vi "tsapp_configure_baudrate_can.vi"(5 "AInstallTermResistor120Ohm":bool, 7 "AListenOnly":bool, 8 "error in (no error)":errorcluster caption="错误输入（无错误）", 9 "ABaudrateKbps":sgl, 10 "AIdxChn":i32, 11 "路径输入":path) -> (0 "error out":errorcluster caption="错误输出", 2 "return":i32, 3 "路径输出":path)   [LabVIEW 2014]
doc: "Function Introduction ：\nSet parameters such as baud rate for CAN channel\nCall location ：\nBefore connecting hardware devices, set the parameters of the channel first\ninput parameter ：\nAIdxChn: Application Channel Number\nABaud rate Kbps: baud rate (kbps)\nAListenOnly: Whether to only listen mode, if enabled, can only receive data\nAInstallTermResistor120Ohm: Can only internal terminal resistors of the device be used\nReturn value ：\n==0: Connection successful\nOther: Check for error codes"
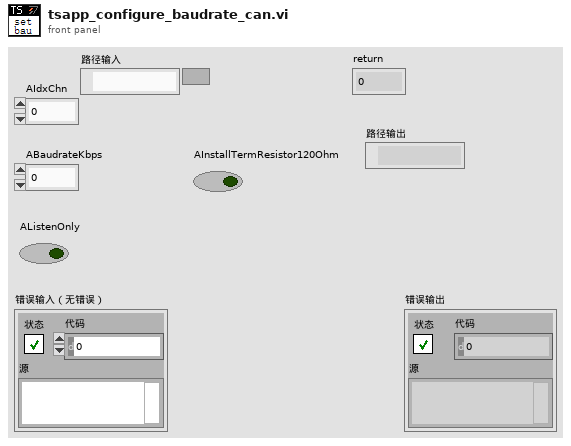
[diagram p1: front panel]
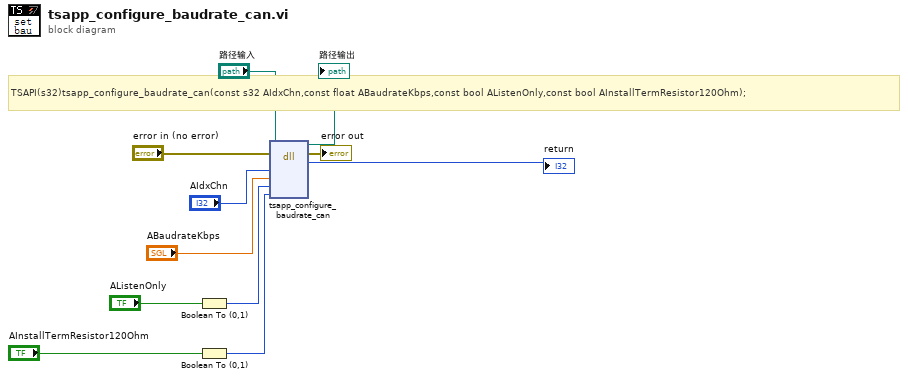
[diagram p0: block diagram]
diagram:
  # "TSAPI(s32)tsapp_configure_baudrate_can(const s32 AIdxChn,const float ABaudrateKbps,const bool AListenOnly,const bool AInstallTermResistor120Ohm);"
  n1 = Boolean To (0,1)(Boolean="AListenOnly") -> (0, 1=w8:i16)
  n2 = Boolean To (0,1)(Boolean="AInstallTermResistor120Ohm") -> (0, 1=w6:i16)
  n3 = dll-call lib="D:/Work/LabVIEW Code/TSMaster Labview SDK/LabVIEW/LabVIEW-TSMasterAPI_CLN/TSMasterAPI_LabVIEW-2024-08-02 09-14-06/Not_organized_vi/TSMaster.*" fn="tsapp_configure_baudrate_can"(path in="路径输入", error in="error in (no error)", "AIdxChn"="AIdxChn", "ABaudrateKbps"="ABaudrateKbps", "AListenOnly"=w8, "AInstallTermResistor120Ohm"=w6) -> (path out=→"路径输出":path, error out=→"error out":errorcluster, "返回类型"=→"return":i32)  [unwired: 5 in]
